vi "LINC Register Handshake.vi"(8 "error in (no error)":errorcluster, 11 "LINC session":refnum<class "LINC.lvclass">) -> (0 "error out":errorcluster, 3 "dup LINC session":refnum<class "LINC.lvclass">)   [LabVIEW 2018, in "STEPkgDriver_LINC.lvlib" / "LINC.lvclass"]
uses:
  LINC.lvclass
  LINC Handshake.ctl
  STEPkgDriver_LINC.lvlib
  LINC Command Origin.ctl
panel:
  in  "HANDSHAKE":T1
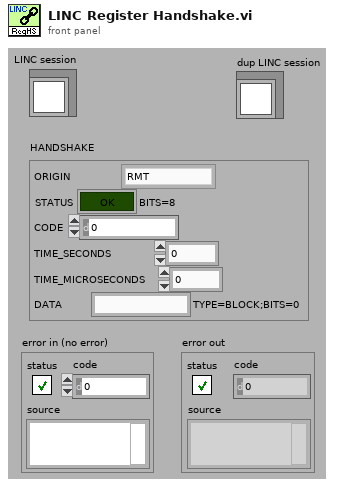
[diagram p1: front panel]
types:
  T1 = typedef "STEPkgDriver_LINC.lvlib/LINC Handshake.ctl" = cluster{"ORIGIN":T2, "STATUS":bool, "CODE":i32, "TIME_SECONDS":u32, "TIME_MICROSECONDS":u32, "DATA":string}
  T2 = typedef "STEPkgDriver_LINC.lvlib/LINC Command Origin.ctl" = enum8{"RMT", "LCL"}
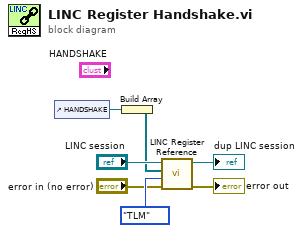
[diagram p0: block diagram]
diagram:
  n1 = control-ref of="HANDSHAKE"() -> (w3:refnum<vi>)
  n2 = Build Array(w3) -> (w5:refnum<vi>[])
  n3 = call "LINC Register Reference.vi"("error in (no error)"="error in (no error)", "type (CMD)"=enum16{"CMD", "TLM", "CMD_HDR", "TLM_HDR"}."TLM", "controls"=w5, "LINC session"="LINC session") -> ("error out"=→"error out":errorcluster, "dup LINC session"=→"dup LINC session":refnum<class "LINC.lvclass">)  [unwired: 6 in]
